vi "Get IC.vi"(8 "error in (no error)":errorcluster, 10 "Domain":refnum<class "NI_Domain.lvclass">, 11 "IC in":refnum<class "NI_IC.lvclass">) -> (0 "error out":errorcluster, 2 "IC":variant, 3 "IC out":refnum<class "NI_IC.lvclass">)   [LabVIEW 2017, in "NI_PDE.lvlib" / "NI_IC.lvclass"]
uses:
  <vilib>/gmath/pde.llb/ICClass/NI_IC.lvclass
  <vilib>/gmath/pde.llb/DomainClass/NI_Domain.lvclass
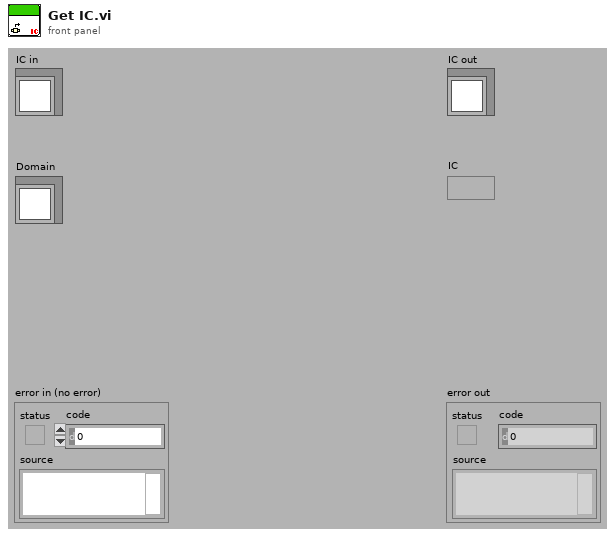
[diagram p1: front panel]
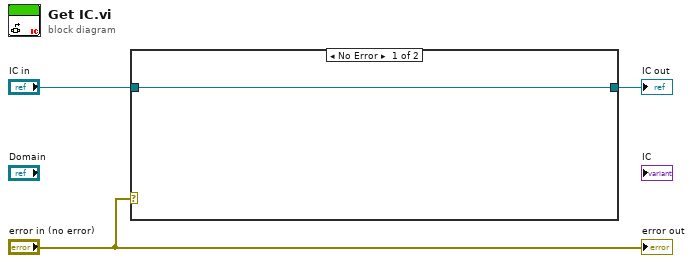
[diagram p0: block diagram]
diagram:
  n1 = case shown="No Error" "error in (no error)" {
    tunnel: "IC in" -> [w4 w5]
    tunnel: [w4 w5] -> w2
    frame No Error {
    }
    frame Error {
    }
  }
  "IC out" <- w2
  "error out" <- "error in (no error)"
